vi "Get Number of Global Teardown Calls.vi"(8 "error in (no error)":errorcluster) -> (0 "error out":errorcluster, 2 "Calls to Teardown":i32)   [LabVIEW 2020, in "Global Fixture Test Double.lvclass"]
uses:
  Global Variable.vi
  Global Fixture Test Double.lvclass
  Global Fixture Test Double.lvclass/Global Fixture Test Double.ctl
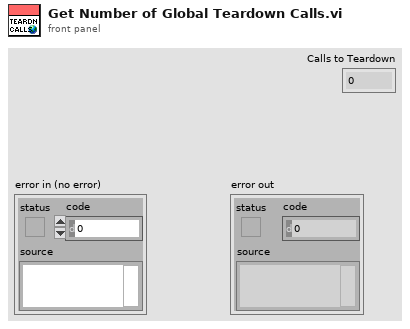
[diagram p1: front panel]
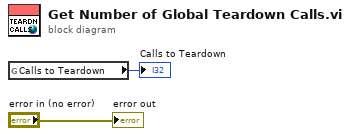
[diagram p0: block diagram]
diagram:
  n1 = global read "Global Variable.vi" "Calls to Teardown"() -> (→"Calls to Teardown":i32)
  "error out" <- "error in (no error)"
